vi "VL Type.vi"(8 "error in (no error)":errorcluster, 11 "State Config in":refnum<class "State Config.lvclass">) -> (0 "error out":errorcluster, 2 "VL Type":T1, 3 "State Config out":refnum<class "State Config.lvclass">)   [LabVIEW 2020, in "VolatusSeqConfig.lvlib" / "State Config.lvclass"]
uses:
  State Config.lvclass
  State Config.lvclass/State Config.ctl
  VolatusConfig/Meta Type.ctl
  VolatusConfig/VolatusConfig.lvlib
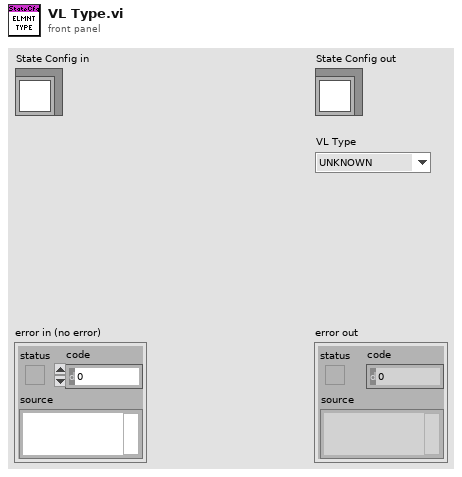
[diagram p1: front panel]
types:
  T1 = typedef "VolatusConfig.lvlib/Meta Type.ctl" = enum16{"UNKNOWN", "VL_System", "VL_Cluster", "VL_Node", "VL_Task", "VL_Group", "VL_Channel", "VL_Task_List", "VL_Scaling", "VL_Sensor", "VL_Sensor_List", "VL_Scale"}
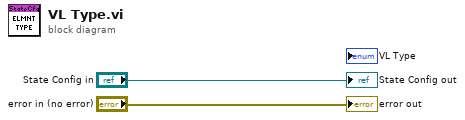
[diagram p0: block diagram]
diagram:
  "error out" <- "error in (no error)"
  "State Config out" <- "State Config in"
